vi "FMV - get cluster details.vi"(8 "error in (no error)":errorcluster, 11 "JSON string":string) -> (0 "error out":errorcluster, 3 "value":string)   [LabVIEW 2020, in "ui-testing.lvlib"]
doc: "copyright: Thomas Zilliox©"
uses:
  ui-testing.lvlib
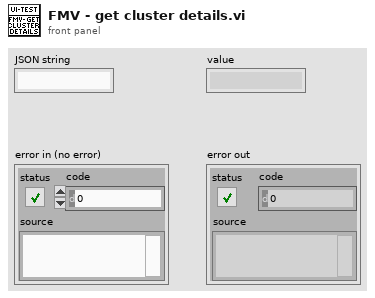
[diagram p1: front panel]
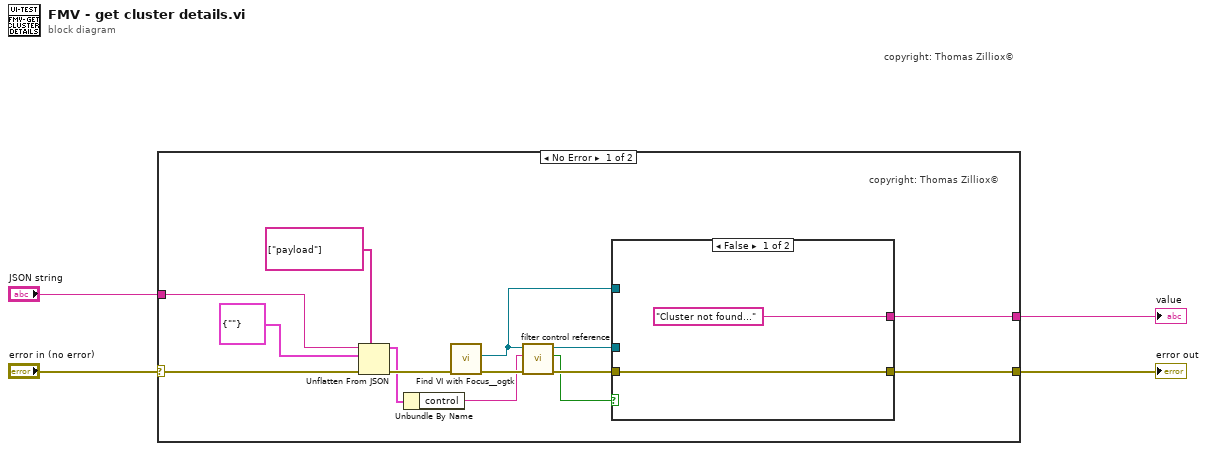
[diagram p0: block diagram]
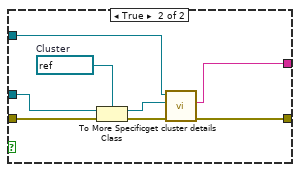
[diagram p2: hidden frame]
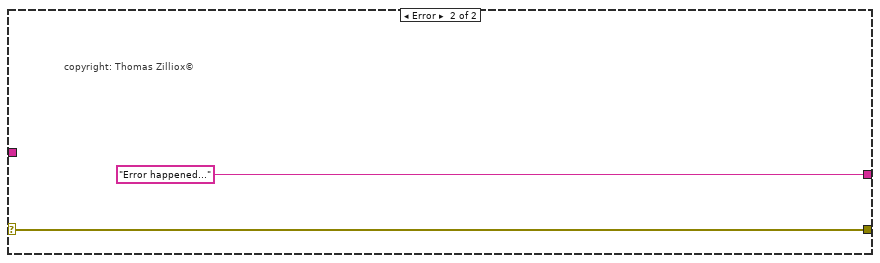
[diagram p3: hidden frame]
diagram:
  # "copyright: Thomas Zilliox©"
  n1 = case shown="No Error" "error in (no error)" {
    selector: "error in (no error)" -> [w16 w30]
    tunnel: "JSON string" -> [w17 _]
    tunnel: [w7 w30] -> w3
    tunnel: [w8 "Error happened..."] -> w2
    frame No Error {
      # "copyright: Thomas Zilliox©"
      n2 = Unflatten From JSON(path=string[] ["payload"], JSON string=w17, type and defaults=cluster{"control":string} {"control"=""}, error in (no error)=w16) -> (value=w6:cluster{"control":string}, error out=w15:errorcluster)  [unwired: 3 in]
      n3 = Unbundle By Name(w6) -> ("control"=w12:string)
      n4 = call <userlib>:"Find VI with Focus__ogtk.vi"("error in"=w15) -> ("error out"=w13:errorcluster, "VI with Focus"=w5:refnum<vi>)  [unwired: 6 in, 3 out]
      n5 = call "filter control reference.vi"("error in (no error)"=w13, "Control label"=w12, "VI (Caller)"=w5) -> ("error out"=w10:errorcluster, "Control found"=w9:bool, "Control ref"=w11:refnum<vi>)  [unwired: 6 in]
      n6 = case shown="False" w9 {
        tunnel: w11 -> [_ w26]
        tunnel: w10 -> [w20 w28]
        tunnel: [w20 w22] -> w7
        tunnel: ["Cluster not found..." w23] -> w8
        tunnel: w5 -> [_ w21]
        frame False {
        }
        frame True {
          w27 = refnum<vi> refnum  # Cluster
          n7 = To More Specific Class(target class=w27, reference=w26, error in=w28) -> (specific class reference=w25:refnum<vi>, error out=w24:errorcluster)
          n8 = call "get cluster details.vi"("error in"=w24, "Cluster-target"=w25, "VI Refnum"=w21) -> ("error out"=w22:errorcluster, "Control details"=w23:string)  [unwired: 7 in]
        }
      }
    }
    frame Error {
      # "copyright: Thomas Zilliox©"
    }
  }
  "error out" <- w3
  "value" <- w2
